vi "GenCylinder.vi"() -> (3 "SceneObject out":refnum<vi>)   [LabVIEW 2012, in "lv-attitudecontrol.lvlib"]
uses:
  lv-attitudecontrol.lvlib
  Controls/PictureTypes.ctl
  <vilib>/picture/3D Picture Control/NI_3D Picture Control.lvlib
panel:
  # "Generates the rotating drum with the picture \nat the path specified below"
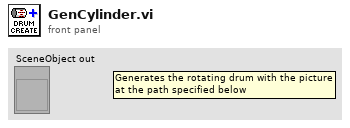
[diagram p1: front panel]
types:
  T1 = typedef "lv-attitudecontrol.lvlib/PictureTypes.ctl" = enum16{"Fixed Horizon", "Altitude Lines", "Dial"}
  T2 = enum16{"Inherit Value", "No Culling", "Cull Back Face", "Cull Front Face", "Cull Both Faces"}
  T3 = enum16{"No Filtration", "Linear Filtration", "Simple Mipmap Filtration", "Bilinear Filtration", "Trilinear Filtration"}
  T4 = enum16{"As a Decal", "With Modulation", "With Blending", "As a replacement"}
  T5 = typedef "imagedata.ctl" = cluster{"image type":i32, "image depth":i32, "image":u8[], "mask":u8[], "colors":u32[], "Rectangle":cluster{"left":i16, "top":i16, "right":i16, "bottom":i16}}
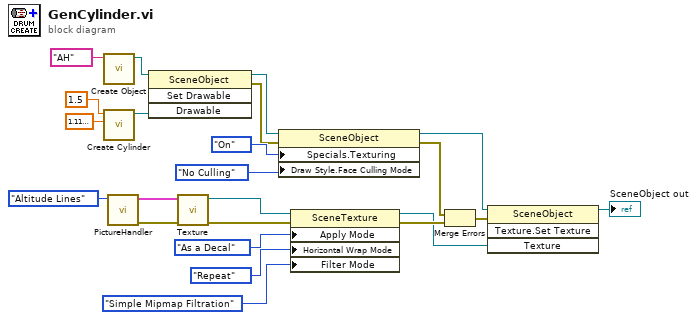
[diagram p0: block diagram]
diagram:
  n1 = call <vilib>:"Create Object.vi"("Name"="AH") -> ("Scene:New Object"=w12:refnum<vi>)  [unwired: 1 in, 9 out]
  n2 = call <vilib>:"Create Cylinder.vi"("Radius"=sgl 1.11 ("Detail"), "Height"=sgl 1.5 ("Radius")) -> ("New Cylinder Refnum"=w8:refnum<vi>)  [unwired: 8 in, 1 out]
  n3 = call "PictureHandler.vi"("Picture"=PictureTypes."Altitude Lines") -> ("error out"=w1:errorcluster, "image data"=w3:T5)  [unwired: 9 in]
  n4 = invoke class="SceneObject" method="Set Drawable"(reference=w12, "Drawable"=w8) -> (reference out=w9:refnum<vi>, error out=w10:errorcluster)  [unwired: 2 in, 2 out]
  n5 = call <vilib>:"Texture.vi"("error in (no error)"=w1, "Image"=w3) -> ("error out"=w20:errorcluster, "New Texture Refnum"=w13:refnum<vi>)  [unwired: 8 in]
  n6 = property class="SceneObject"(reference=w9, error in=w10, "Specials.Texturing"=enum16{"Inherit Value", "Off", "On"}."On" ("Specials:Texturing"), "Draw Style.Face Culling Mode"=T2."No Culling" ("Draw Style:Face Culling Mode")) -> (reference out=w17:refnum<vi>, error out=w21:errorcluster)
  n7 = property class="SceneTexture"(reference=w13, error in=w20, "Apply Mode"=T4."As a Decal", "Horizontal Wrap Mode"=enum16{"Clamp", "Repeat"}."Repeat", "Filter Mode"=T3."Simple Mipmap Filtration") -> (reference out=w18:refnum<vi>, error out=w22:errorcluster)
  n8 = Merge Errors(w21, w22) -> (w19:errorcluster)
  n9 = invoke class="SceneObject" method="Texture.Set Texture"(reference=w17, error in=w19, "Texture"=w18) -> (reference out=→"SceneObject out":refnum<vi>)  [unwired: 1 in, 3 out]
